vi "__initalizeRoomsConfiguration.vi"(8 "error in":errorcluster, 11 "path in":path) -> (0 "error out":errorcluster, 3 "file path out":path)   [LabVIEW 2020, in "Room-API.lvclass"]
uses:
  Room-API.lvclass
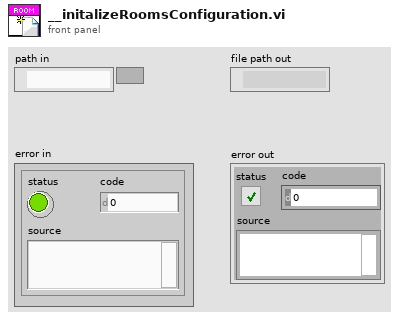
[diagram p1: front panel]
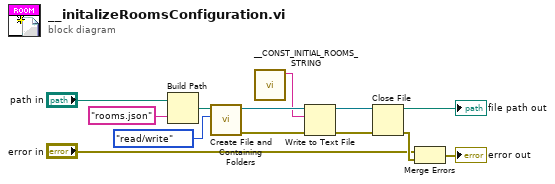
[diagram p0: block diagram]
diagram:
  n1 = Build Path(base path="path in", name or relative path="rooms.json") -> (appended path=w11:path)
  n2 = call <vilib>:"Create File and Containing Folders.vi"("access"=enum16{"read/write", "read-only", "write-only"}."read/write", "file path"=w11) -> ("error out"=w6:errorcluster, "refnum out"=w12:refnum<file>)  [unwired: 8 in]
  n3 = call "__CONST_INITIAL_ROOMS_STRING.vi"() -> ("inital rooms text"=w4:string)  [unwired: 11 in]
  n4 = Write to Text File(file (use dialog)=w12, text=w4, error in=w6) -> (refnum out=w7:refnum<file>, error out=w5:errorcluster)  [unwired: 1 in, 1 out]
  n5 = Close File(refnum=w7, error in=w5) -> (path=→"file path out":path, error out=w3:errorcluster)
  n6 = Merge Errors("error in", w3) -> (→"error out":errorcluster)
